vi "Get Channel Version.vi"(0 "VISA Session In":refnum<visa-resource-name>="OXYMAT", 1 "Target Address":u8=16 format="%.0x", 2 "Source Address":u8=208 format="%.0x", 11 "error in (no error)":errorcluster) -> (4 "VISA Session Out":refnum<visa-resource-name>, 6 "Message Header":T2 {"Source Address" format="%.0x"; "Target Address" format="%.0x"}, 8 "Channel Type":T4(ring), 10 "Channel":T1, 13 "Success":bool, 15 "error out":errorcluster)   [LabVIEW 2023, in "Siemens ELAN.lvlib"]
doc: "Using the Siemens ELAN protocol, gets version information from the addressed analyzer. Also returns a boolean indicating that the addressed device provided a valid response.\n\n$Revision:: 0 $\n$Modtime:: yy-mm-dd hh:mm $\n$Author:: Dboyd $"
uses:
  Siemens ELAN.lvlib
  Message Header.ctl
  Channel Status.ctl
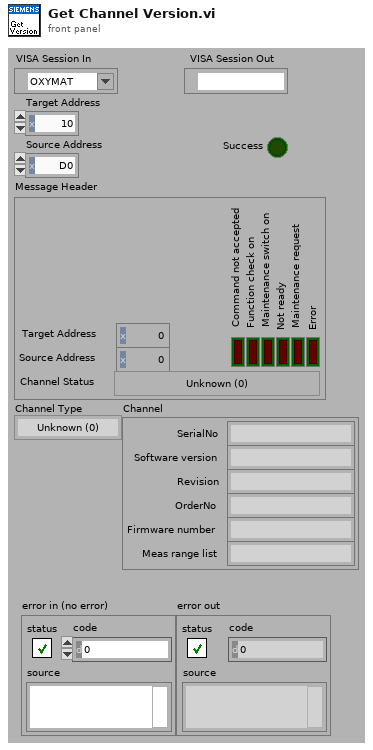
[diagram p1: front panel]
types:
  T1 = cluster{"SerialNo":string, "Software version":string, "Revision":string, "OrderNo":string, "Firmware number":string, "Meas range list":string}
  T2 = typedef "Siemens ELAN.lvlib/Message Header.ctl" = cluster{"Target Address":u8, "Source Address":u8, "Error":bool, "Maintenance request":bool, "Not ready":bool, "Maintenance switch on":bool, "Function check on":bool, "Command not accepted":bool, "Channel Status":T3}
  T3 = typedef "Siemens ELAN.lvlib/Channel Status.ctl" = enum8{"Unknown (0)", "Warm-up", "Pause", "Standby", "Measure", "Zero calibration", "Adjust component slope", "Unknown (7)", "Adjust curve dip", "Adjust linearization sensitivity", "Adjust temperature compensation", "Adjust pressure compensation", "Adjust linearization zero", "Adjust flow sensor", "Autocal", "Adjust phase", "Zero calibration of O2 sensor", "Synchronous zero calibration", "Purging for synchronous zero calibration", "Adjust analog output", "Adjust analog input", "Cleaning", "Unknown (>21)"}
  T4 = enum8{"Unknown (0)", "ULTRAMAT 6", "OXYMAT 6", "FIDAMAT 6", "ULTRAMAT 23", "SIPAN 34", "Unknown (6)", "CALOMAT 6", "Unknown (>7)"}
  T5 = cluster{"[0]":string, "[1]":string, "[2]":string, "[3]":string, "[4]":string, "[5]":string}
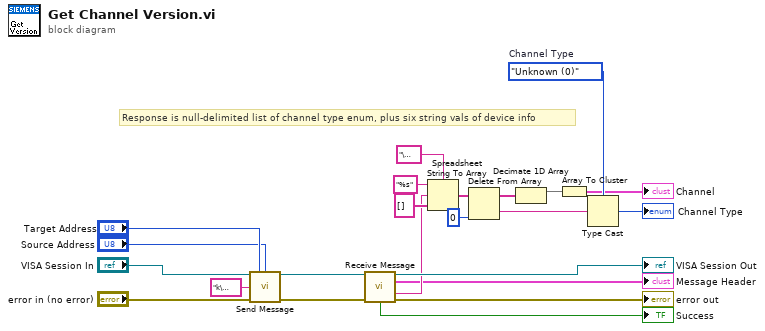
[diagram p0: block diagram]
diagram:
  w5 = T4."Unknown (0)"  # Channel Type
  # "Response is null-delimited list of channel type enum, plus six string vals of device info"
  n1 = call "Send Message.vi"("VISA Session In"="VISA Session In", "Target Address"="Target Address", "Source Address"="Source Address", "Command"="k\u0006", "error in (no error)"="error in (no error)") -> ("VISA Session Out"=w23:refnum<visa-resource-name>, "error out"=w22:errorcluster)  [unwired: 8 in, 1 out]
  n2 = call "Receive Message.vi"("VISA Session In"=w23, "error in (no error)"=w22) -> ("VISA Session Out"=→"VISA Session Out":refnum<visa-resource-name>, "Message Header"=→"Message Header":T2, "Response"=w13:string, "Success"=→"Success":bool, "error out"=→"error out":errorcluster)  [unwired: 8 in, 1 out]
  n3 = Spreadsheet String To Array(delimiter (Tab)="\u0000", format string="%s", spreadsheet string=w13, array type (2D Dbl)=string[] []) -> (array=w10:string[])
  n4 = Delete From Array(array=w10, index=0) -> (deleted portion=w6:string, array with subset deleted=w2:string[])  [unwired: 1 in]
  n5 = Decimate 1D Array(w2) -> (w1:string[])  [unwired: 1 out]
  n6 = Array To Cluster(array=w1) -> (cluster=→"Channel":T5)
  n7 = Type Cast(type=w5, x=w6) -> (*(type *) &x=→"Channel Type":T4)
